vi "HexStr2StrU8.vi"(11 "HEX文字列":string) -> (1 "string":string, 3 "U8[]":u8[](array[numeric]) format="%.0x")   [LabVIEW 2014]
panel:
  # "C0 FF 01 ･･･"
  # "16進、区切りスペースの文字列"
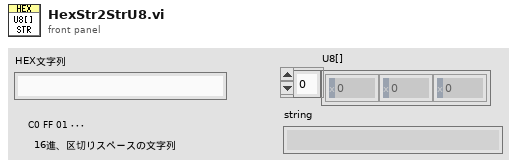
[diagram p1: front panel]
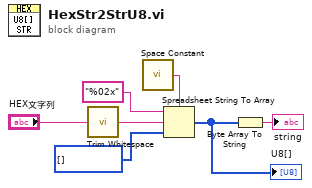
[diagram p0: block diagram]
diagram:
  n1 = call <vilib>:"Trim Whitespace.vi"("string"="HEX文字列") -> ("trimmed string"=w2:string)  [unwired: 1 in]
  n2 = call <vilib>:"Space Constant.vi"() -> ("String"=w1:string)
  n3 = Spreadsheet String To Array(delimiter (Tab)=w1, format string="%02x" ("形式文字列"), spreadsheet string=w2, array type (2D Dbl)=u8[] []) -> (array=w3:u8[])
  "U8[]" <- w3
  n4 = Byte Array To String(unsigned byte array=w3) -> (string=→"string":string)
